vi "Format Helium Test Result Table.vi"(10 "Test Config":T1, 11 "Test Results":T7) -> (2 "Failure Indexes":i32[](array[numeric]), 3 "Helium Results":string[][](array[string]))   [LabVIEW 2014]
uses:
  Tests/Controls/Test Results.ctl
  Tests/Controls/Step Result.ctl
  Tests/Controls/Test Information.ctl
  Tests/Controls/Vacuum Test.ctl
  Tests/Controls/Test Timing.ctl
  Tests/Controls/Vaccum Thresholds.ctl
  Tests/Controls/Helium Test.ctl
  Tests/Controls/Helium Thresholds.ctl
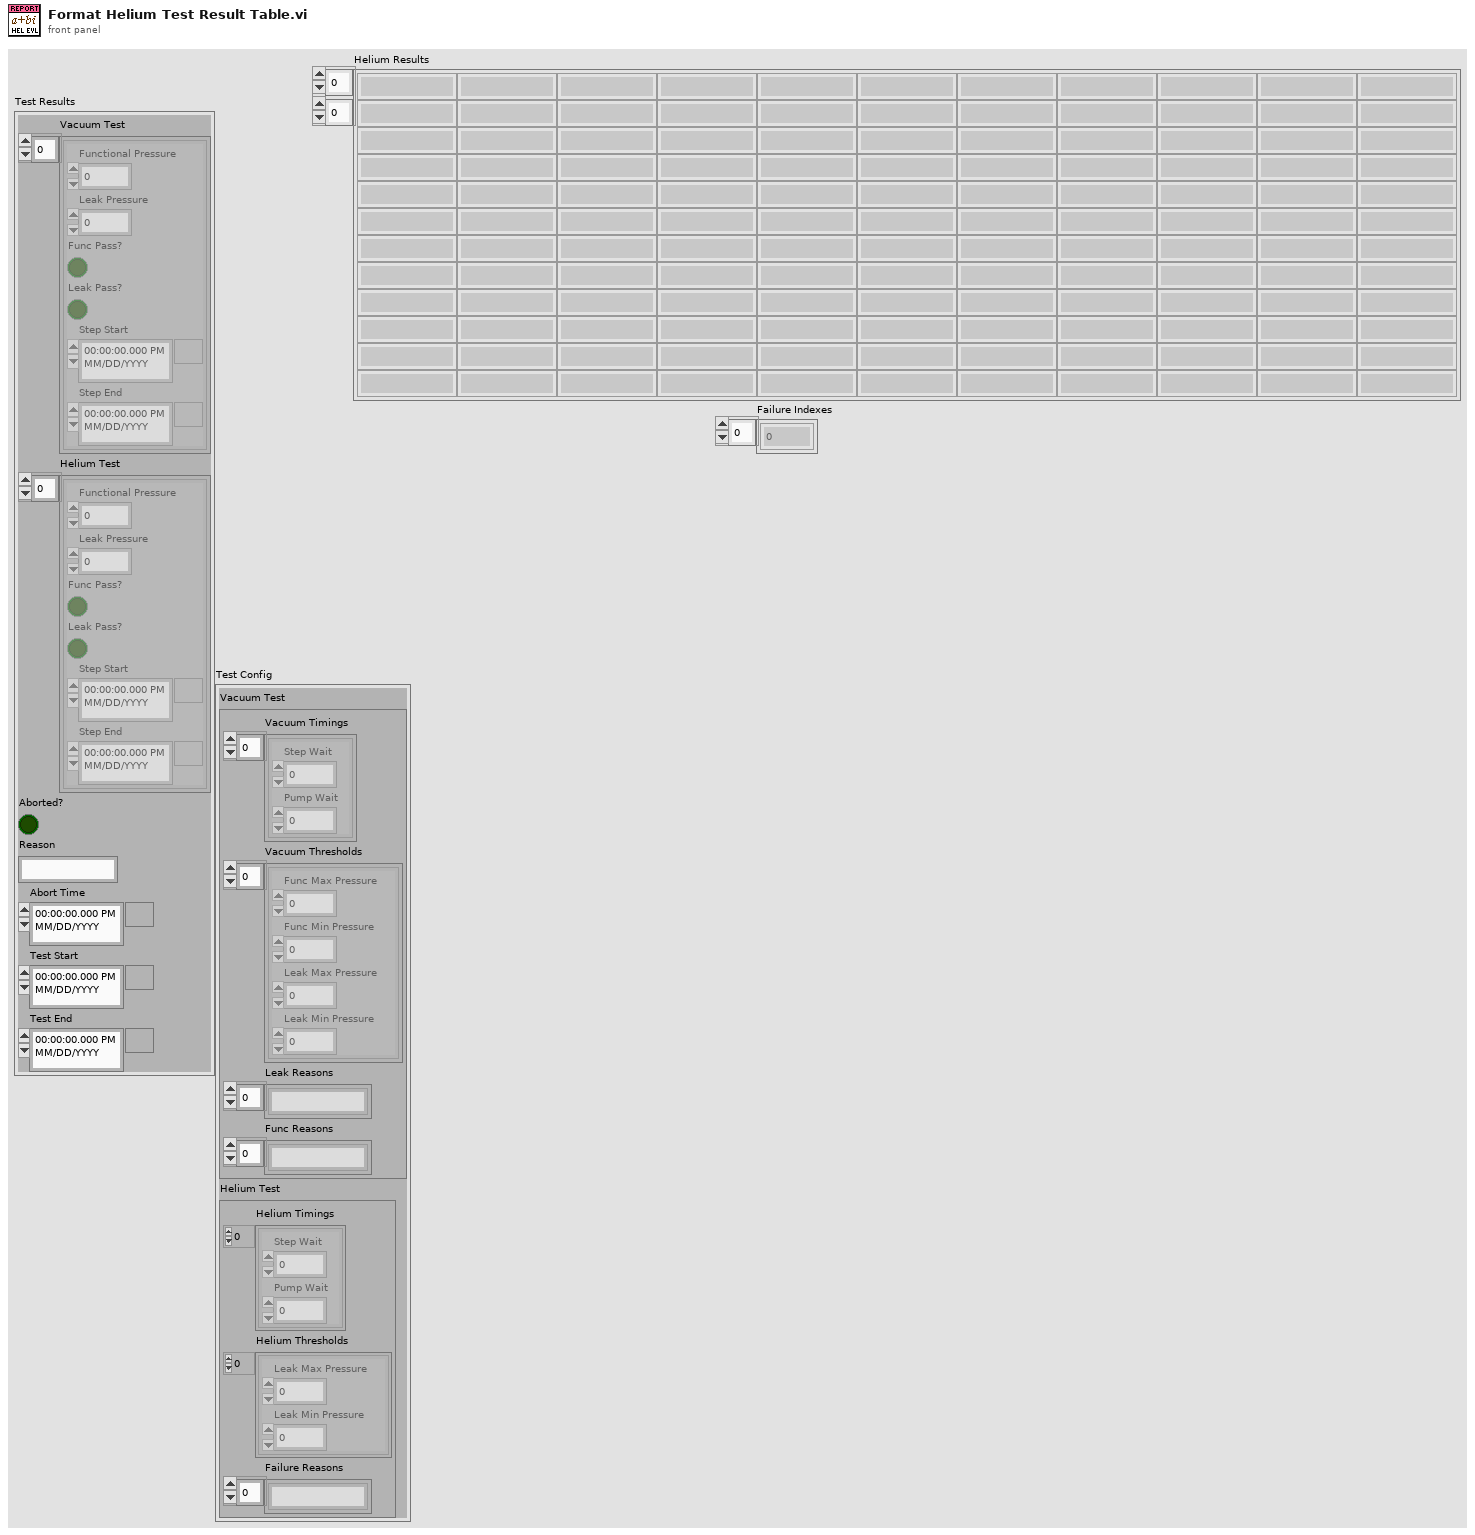
[diagram p1: front panel]
types:
  T1 = typedef "Test Information.ctl" = cluster{"Vacuum Test":T2, "Helium Test":T5}
  T2 = typedef "Vacuum Test.ctl" = cluster{"Vacuum Timings":T3[], "Vacuum Thresholds":T4[], "Leak Reasons":string[], "Func Reasons":string[]}
  T3 = typedef "Test Timing.ctl" = cluster{"Step Wait":dbl, "Pump Wait":dbl}
  T4 = typedef "Vaccum Thresholds.ctl" = cluster{"Func Max Pressure":dbl, "Func Min Pressure":dbl, "Leak Max Pressure":dbl, "Leak Min Pressure":dbl}
  T5 = typedef "Helium Test.ctl" = cluster{"Helium Timings":T3[], "Helium Thresholds":T6[], "Failure Reasons":string[]}
  T6 = typedef "Helium Thresholds.ctl" = cluster{"Leak Max Pressure":dbl, "Leak Min Pressure":dbl}
  T7 = typedef "Test Results.ctl" = cluster{"Vacuum Test":T8[], "Helium Test":T8[], "Aborted?":bool, "Reason":string, "Abort Time":timestamp, "Test Start":timestamp, "Test End":timestamp}
  T8 = typedef "Step Result.ctl" = cluster{"Functional Pressure":dbl, "Leak Pressure":dbl, "Func Pass?":bool, "Leak Pass?":bool, "Step Start":timestamp, "Step End":timestamp}
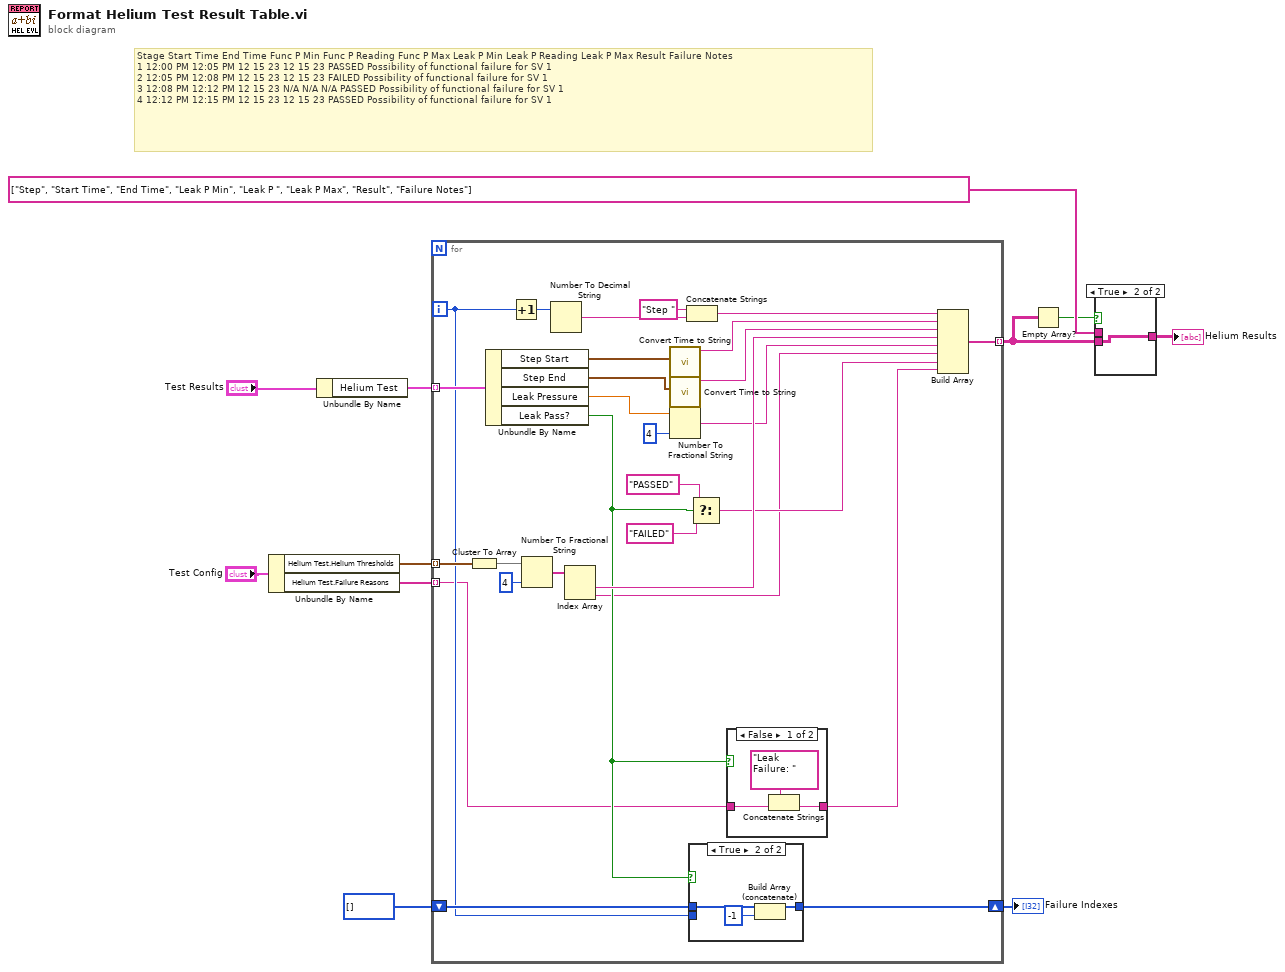
[diagram p0: block diagram]
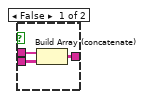
[diagram p2: hidden frame]
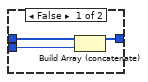
[diagram p3: hidden frame]
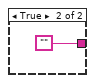
[diagram p4: hidden frame]
diagram:
  # "Stage\tStart Time\tEnd Time\tFunc P Min\tFunc P Reading\tFunc P Max\tLeak P Min\tLeak P Reading\tLeak P Max\tResult\tFailure Notes\n1\t12:00 PM\t12:05 PM\t12\t15\t23\t12\t15\t23\tPASSED\tPossibility of functional failure for SV 1\n2\t12:05 PM\t12:08 PM\t12\t15\t23\t12\t15\t23\tFAILED\tPossibility of functional failure for SV 1\n3\t12:08 PM\t12:12 PM\t12\t15\t23\tN/A\tN/A\tN/A\tPASSED\tPossibility of functional failure for SV 1\n4\t12:12 PM\t12:15 PM\t12\t15\t23\t12\t15\t23\tPASSED\tPossibility of functional failure for SV 1"
  n1 = Unbundle By Name("Test Config") -> ("Helium Test.Helium Thresholds"=w8:T6[], "Helium Test.Failure Reasons"=w7:string[])
  n2 = Unbundle By Name("Test Results") -> ("Helium Test"=w10:T8[])
  n3 = for {
    tunnel: w10 -> [w39] mode=indexing
    tunnel: w8 -> [w35] mode=indexing
    tunnel: w7 -> [w12] mode=indexing
    tunnel: [w20] -> w2 mode=indexing
    shift-right: [w17] -> w3
    shift-left: i32[] [] -> [w19]
    i -> [w18]
    n4 = Cluster To Array(cluster=w35) -> (array=w34:dbl[])
    n5 = Unbundle By Name(w39) -> ("Step Start"=w37:timestamp, "Step End"=w36:timestamp, "Leak Pressure"=w24:dbl, "Leak Pass?"=w16:bool)
    n6 = Increment(x=w18) -> (x+1=w38:i32)
    n7 = Number To Fractional String(number=w34, precision (6)=i16 4) -> (F-format string=w32:string[])  [unwired: 2 in]
    n8 = Number To Decimal String(number=w38) -> (decimal integer string=w31:string)  [unwired: 1 in]
    n9 = Index Array(array=w32) -> (element #1=w26:string, element #2=w14:string)  [unwired: 2 in]
    n10 = call "Convert Time to String.vi"("time stamp"=w37) -> ("date/time string"=w28:string)  [unwired: 10 in]
    n11 = call "Convert Time to String.vi"("time stamp"=w36) -> ("date/time string"=w27:string)  [unwired: 10 in]
    n12 = Number To Fractional String(number=w24, precision (6)=i16 4) -> (F-format string=w15:string)  [unwired: 2 in]
    n13 = Concatenate Strings("Step " ("string"), w31) -> (w30:string)
    n14 = case shown="True" w16 {
      tunnel: w19 -> [w42 w45]
      tunnel: w18 -> [w41 _]
      tunnel: [w40 w44] -> w17
      frame False {
        n15 = Build Array (concatenate)(w42, w41) -> (w40:i32[])
      }
      frame True {
        n16 = Build Array (concatenate)(w45, -1) -> (w44:i32[])
      }
    }
    n17 = Select(t="PASSED", s=w16, f="FAILED") -> (s? t:f=w21:string)
    n18 = case shown="False" w16 {
      tunnel: [w47 ""] -> w13
      tunnel: w12 -> [w48 _]
      frame False {
        n19 = Concatenate Strings("Leak Failure: " ("string"), w48) -> (w47:string)
      }
      frame True {
      }
    }
    n20 = Build Array(w30, w28, w27, w26, w15, w14, w21, w13) -> (w20:string[])
  }
  "Failure Indexes" <- w3
  n21 = Empty Array?(array=w2) -> (empty?=w1:bool)
  n22 = case shown="True" w1 {
    tunnel: string[] ["Step", "Start Time", "End Time", "Leak P Min", "Leak P ", "Leak P Max", "Result", "Failure Notes"] -> [w52 _]
    tunnel: [w51 w53] -> w5
    tunnel: w2 -> [w50 w53]
    frame False {
      n23 = Build Array (concatenate)(w52, w50) -> (w51:string[][])
    }
    frame True {
    }
  }
  "Helium Results" <- w5
